vi "Condition Type.vi"(11 "LowLimit Condition Config in":refnum<class "LowLimit Condition Config.lvclass">) -> (2 "Condition Type":string)   [LabVIEW 2020, in "VolatusSeqConfig.lvlib" / "LowLimit Condition Config.lvclass"]
uses:
  LowLimit Condition Config.lvclass
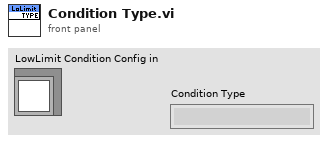
[diagram p1: front panel]
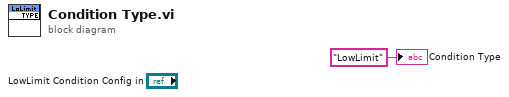
[diagram p0: block diagram]
diagram:
  "Condition Type" <- "LowLimit" ("Condition Type")
